vi "Init Tree.vi"(8 "error in":errorcluster) -> (0 "error out":errorcluster, 3 "Tree Map out":refnum<class "Tree Map.lvclass">)   [LabVIEW 2023, in "VI Properties Editor.lvlib"]
uses:
  VI Properties Editor.lvlib
  Tree Map/Tree Map/Tree Map.lvclass
  CTLs/Custom Symbols.ctl
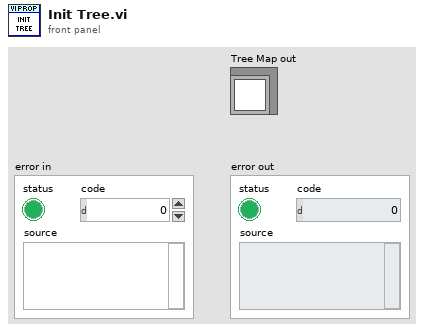
[diagram p1: front panel]
types:
  T1 = typedef "VI Properties Editor.lvlib/Custom Symbols.ctl" = cluster{"Symbol Paths":path[], "IDs":string[]}
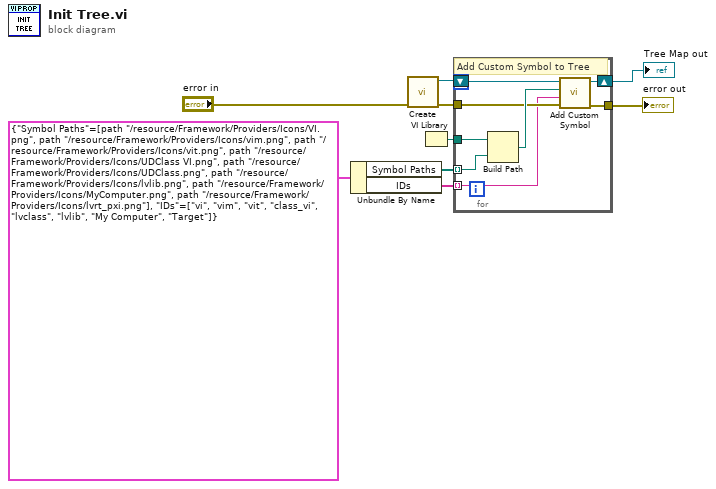
[diagram p0: block diagram]
diagram:
  n1 = Unbundle By Name(T1 {"Symbol Paths"=[path "../resource/Framework/Providers/Icons/VI.png", path "../resource/Framework/Providers/Icons/vim.png", path "../resource/Framework/Providers/Icons/vit.png", path "../resource/Framework/Providers/Icons/UDClass VI.png", path "../resource/Framework/Providers/Icons/UDClass.png", path "../resource/Framework/Providers/Icons/lvlib.png", path "../resource/Framework/Providers/Icons/MyComputer.png", path "../resource/Framework/Providers/Icons/lvrt_pxi.png"], "IDs"=["vi", "vim", "vit", "class_vi", "lvclass", "lvlib", "My Computer", "Target"]} ("Custom Symbols")) -> ("Symbol Paths"=w8:path[], "IDs"=w7:string[])
  n2 = call "Create.vi"("error in (no error)"="error in") -> ("error out"=w2:errorcluster, "Tree Map out"=w1:refnum<class "Tree Map.lvclass">)  [unwired: 9 in]
  n3 = VI Library() -> (path=w6:path)
  n4 = for {
    tunnel: w6 -> [w17]
    shift-right: [w14] -> w3
    shift-left: w1 -> [w16]
    tunnel: w2 -> [w12]
    tunnel: [w13] -> w5
    tunnel: w7 -> [w10] mode=indexing
    tunnel: w8 -> [w11] mode=indexing
    # "Add Custom Symbol to Tree"
    n5 = Build Path(base path=w17, name or relative path=w11) -> (appended path=w15:path)
    n6 = call "Add Custom Symbol.vi"("error in"=w12, "Symbol ID"=w10, "Symbol File Path"=w15, "Tree Map"=w16) -> ("error out"=w13:errorcluster, "Tree Map"=w14:refnum<class "Tree Map.lvclass">)  [unwired: 6 in]
  }
  "error out" <- w5
  "Tree Map out" <- w3
